vi "Camera Interpreter.vi"() -> (0 "error out":errorcluster, 1 "Overhead Image":T4(plugin-control), 2 "Heading":T1 format="%05.1f", 3 "Boat Location":T2, 4 "Time Elapsed (s)\nSince Last Image":dbl)   [LabVIEW 2011]
uses:
  <vilib>/userDefined/High Color/IMAQdx.ctl
  2-RIO/2 Typedefs/UTM Location.ctl
  2-RIO/2 Typedefs/heading.ctl
  <vilib>/vision/driver/NI_Vision_Acquisition_Software.lvlib
panel:
  in  "Reset Camera":bool
  in  "Camera Selector":T3="cam0"
  # "THIS IS A PLACEHOLDER VI\nTHIS IS A PLACEHOLDER VI\nTHIS IS A PLACEHOLDER VI"
  # "(ignore UTM Zone \nand Hemisphere for \nRC boat)"
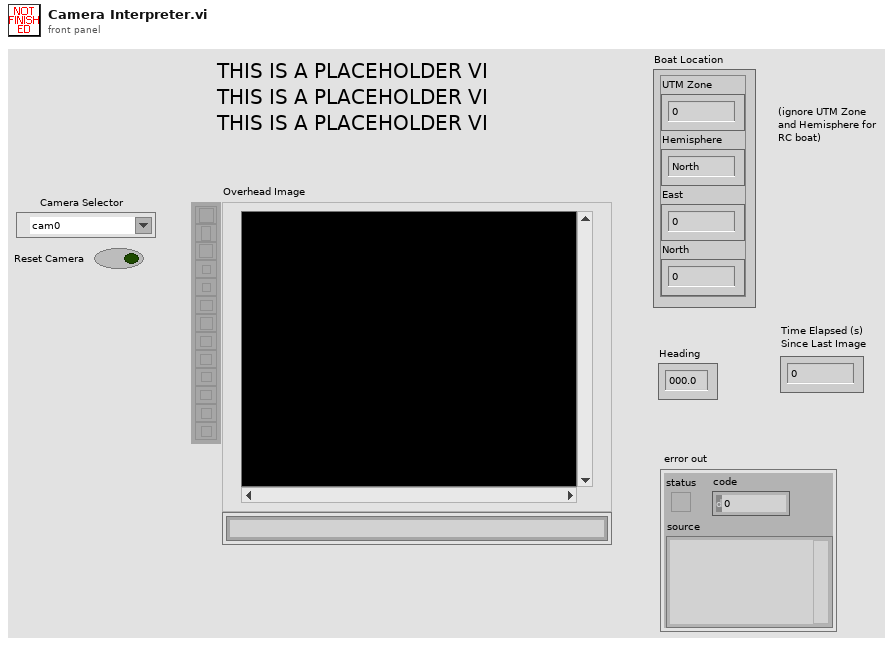
[diagram p1: front panel]
types:
  T1 = typedef "heading.ctl" = dbl
  T2 = typedef "UTM Location.ctl" = cluster{"UTM Zone":dbl, "Hemisphere":enum16{"North", "South"}, "East":dbl, "North":dbl}
  T3 = typedef "IMAQdx.ctl" = refnum<k21>
  T4 = typedef "IMAQ Image.ctl" = refnum<image>
  T5 = typedef "Image Type" = u32
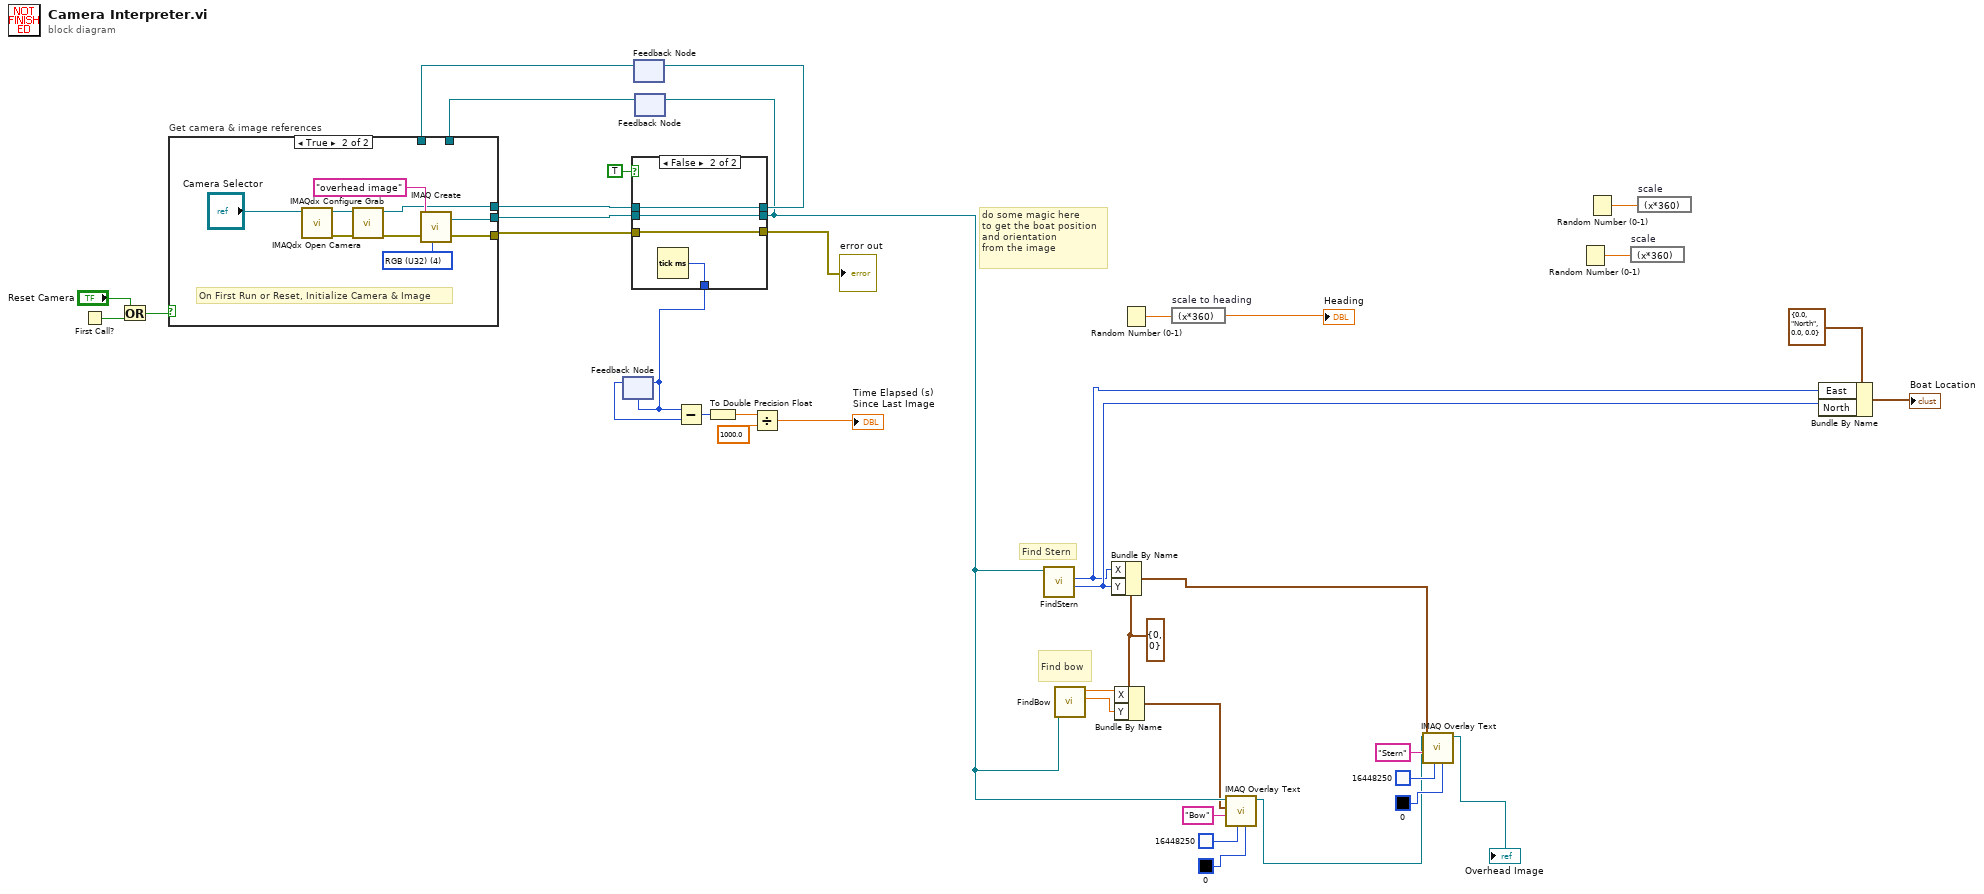
[diagram p0: block diagram]
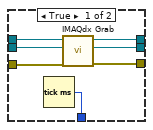
[diagram p2: hidden frame]
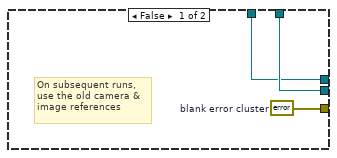
[diagram p3: hidden frame]
diagram:
  w12 = cluster{"X":i32, "Y":i32} {"X"=0, "Y"=0} ("Origin")
  # "Find bow"
  # "Find Stern"
  # "do some magic here\nto get the boat position\nand orientation\nfrom the image"
  n1 = First Call?() -> (First Call?: T/F=w37:bool)
  n2 = Or(x="Reset Camera", y=w37) -> (x .or. y?=w30:bool)
  n3 = feedback #1() -> (w31:T3)  [unwired: 1 in]
  n4 = feedback #2() -> (w32:T4)  [unwired: 1 in]
  n5 = case "Get camera & image references" shown="True" w30 {
    tunnel: [w41 w45] -> w36
    tunnel: [w40 w44] -> w35
    tunnel: [w42 w43] -> w34
    tunnel: w32 -> [w42 _]
    tunnel: w31 -> [w41 _]
    frame False {
      w40 = errorcluster {"status"=FALSE, "code"=0, "source"=""}  # blank error cluster
      # "On subsequent runs,\nuse the old camera &\nimage references"
    }
    frame True {
      w47 = T5 4 items=["Grayscale (U8)", "Grayscale (I16)", "Grayscale (SGL)", "Complex (CSG)", "RGB (U32)", "HSL (U32)", "RGB (U64)", "Grayscale (U16)"] ("Image Type")
      # "On First Run or Reset, Initialize Camera & Image"
      n6 = call <vilib>:"IMAQdx Open Camera.vi"("Session In"="Camera Selector") -> ("error out"=w48:errorcluster, "Session Out"=w51:T3)  [unwired: 9 in]
      n7 = call <vilib>:"IMAQdx Configure Grab.vi"("error in"=w48, "Session In"=w51) -> ("error out"=w49:errorcluster, "Session Out"=w45:T3)  [unwired: 8 in]
      n8 = call "IMAQ Create"("Image Name"="overhead image", "Image Type"=w47, "error in (no error)"=w49) -> ("New Image"=w43:T4, "error out"=w44:errorcluster)  [unwired: 2 in]
    }
  }
  n9 = case shown="False" TRUE {
    tunnel: [w58 w60] -> w38
    tunnel: w36 -> [w57 w62]
    tunnel: w35 -> [w56 w60]
    tunnel: w34 -> [w55 w61]
    tunnel: [w54 w61] -> w10
    tunnel: [w53 w62] -> w33
    tunnel: [w52 w59] -> w21
    frame True {
      n10 = Tick Count (ms)() -> (millisecond timer value=w52:u32)
      n11 = call <vilib>:"IMAQdx Grab.vi"("error in"=w56, "Image In"=w55, "Session In"=w57) -> ("error out"=w58:errorcluster, "Image Out"=w54:T4, "Session Out"=w53:T3)  [unwired: 5 in, 1 out]
    }
    frame False {
      n12 = Tick Count (ms)() -> (millisecond timer value=w59:u32)
    }
  }
  "error out" <- w38
  n13 = feedback-in #3(w21) -> ()
  n14 = feedback #3(w21) -> (w26:u32)
  n15 = feedback-in #1(w33) -> ()
  n16 = feedback-in #2(w10) -> ()
  n17 = Subtract(x=w21, y=w26) -> (x-y=w25:u32)
  n18 = To Double Precision Float(number=w25) -> (double precision float=w24:dbl)
  n19 = Divide(x=w24, y=1000.0) -> (x/y=→"Time Elapsed (s)\nSince Last Image":dbl)
  n20 = call "FindStern.vi"("Refnum in"=w10) -> ("y pixel"=w14:i32, "x pixel"=w13:i32)  [unwired: 7 in, 2 out]
  n21 = call "FindBow.vi"("Refnum in"=w10) -> ("bow pixel y"=w15:sgl, "bow pixel x"=w16:sgl)  [unwired: 7 in, 2 out]
  n22 = Bundle By Name(cluster=w12, "X"=w13, "Y"=w14) -> (w1:cluster{"X":i32, "Y":i32})
  n23 = Bundle By Name(cluster=w12, "X"=w16, "Y"=w15) -> (w9:cluster{"X":i32, "Y":i32})
  n24 = Random Number (0-1)() -> (number: 0 to 1=w39:dbl)
  n25 = expression code="(x*360)" "scale to heading"(w39) -> (→"Heading":dbl)
  n26 = call "IMAQ Overlay Text"("BG Color (Transparent)"=u32 0, "Text Color (black)"=u32 16448250, "String"="Bow", "Origin"=w9, "Image"=w10) -> ("Image Out"=w3:T4)  [unwired: 5 in, 1 out]
  n27 = call "IMAQ Overlay Text"("BG Color (Transparent)"=u32 0, "Text Color (black)"=u32 16448250, "String"="Stern", "Origin"=w1, "Image"=w3) -> ("Image Out"=→"Overhead Image":T4)  [unwired: 5 in, 1 out]
  n28 = Random Number (0-1)() -> (number: 0 to 1=w19:dbl)
  n29 = Random Number (0-1)() -> (number: 0 to 1=w18:dbl)
  n30 = expression code="(x*360)" "scale"(w19) -> ()  [unwired: 1 out]
  n31 = expression code="(x*360)" "scale"(w18) -> ()  [unwired: 1 out]
  n32 = Bundle By Name(cluster=T2 {"UTM Zone"=0.0, "Hemisphere"=enum."North", "East"=0.0, "North"=0.0} ("UTM Location 2"), "East"=w13, "North"=w14) -> (→"Boat Location":T2)
